vi "Value String to Details.vi"(9 "Datatype":T1, 10 "Default":variant, 11 "Value String":string) -> (2 "Identified?":bool, 3 "Value Variant":variant)   [LabVIEW 2016]
uses:
  data types/Datatype.ctl
  <userlib>/_OpenG.lib/lvdata/lvdata.llb/Type Descriptor Enumeration__ogtk.ctl
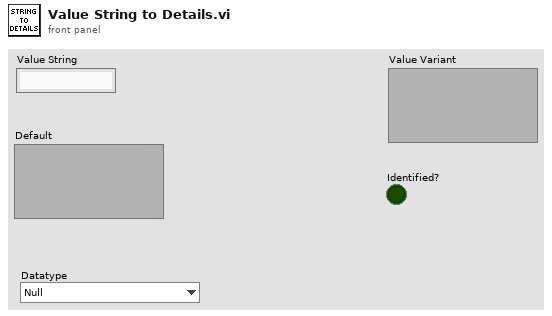
[diagram p1: front panel]
types:
  T1 = typedef "Datatype.ctl" = enum16{"Null", "Numeric", "String", "Bool", "Numeric 1D", "String 1D", "Bool 1D", "Numeric 2D", "String 2D", "Bool 2D", "Variant"}
  T2 = typedef "Type Descriptor Enumeration__ogtk.ctl" = enum8{"<Null>", "I8", "I16", "I32", "I64", "U8", "U16", "U32", "U64", "SGL", "DBL", "EXT", "CSG", "CDB", "CXT", "0x0F", "0x10", "0x11", "0x12", "0x13", "0x14", "Enum U8", "Enum U16", "Enum U32", "Enum U64", "SGL PQ", "DBL PQ", "EXT PQ", "CSG PQ", "CDB PQ", "CXT PQ", "0x1F", "0x20", "Boolean", "0x22", "0x23", "0x24", "0x25", "0x26", "0x27", "0x28", "0x29", "0x2A", "0x2B", "0x2C", "0x2D", "0x2E", "0x2F", "String", "0x31", "Path", "Pict", "0x34", "0x35", "0x36", "DAQ", "0x38", "0x39", "0x3A", "0x3B", "0x3C", "0x3D", "0x3E", "0x3F", "Array", "0x41", "0x42", "0x43", "0x44", "0x45", "0x46", "0x47", "0x48", "0x49", "0x4A", "0x4B", "0x4C", "0x4D", "0x4E", "0x4F", "Cluster", "0x51", "0x52", "Variant", "Waveform", "0x55", "0x56", "0x57", "0x58", "0x59", "0x5A", "0x5B", "0x5C", "0x5D", "0x5E", "0x5F", "0x60", "0x61", "0x62", "0x63", "0x64", "0x65", "0x66", "0x67", "0x68", "0x69", "0x6A", "0x6B", "0x6C", "0x6D", "0x6E", "0x6F", "Refnum"}
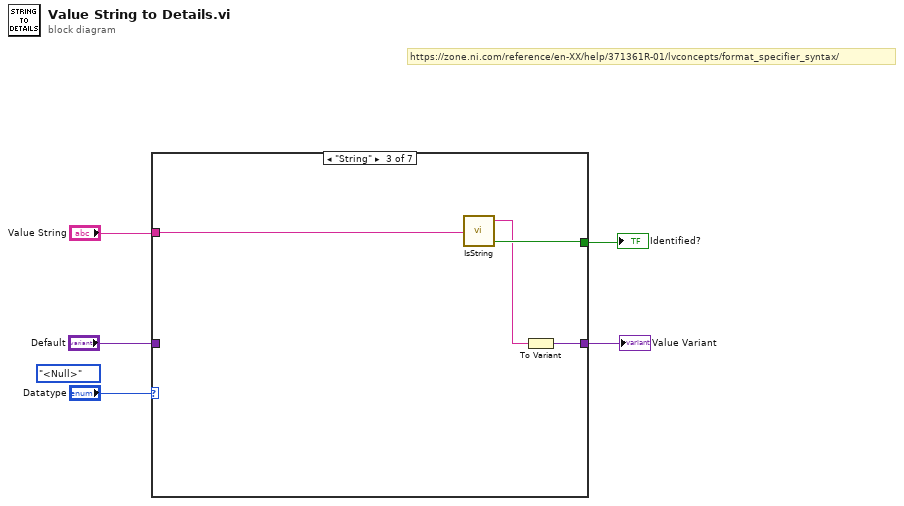
[diagram p0: block diagram]
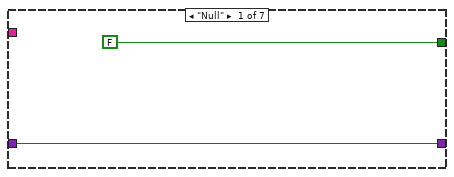
[diagram p2: hidden frame]
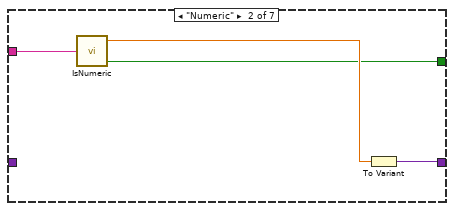
[diagram p3: hidden frame]
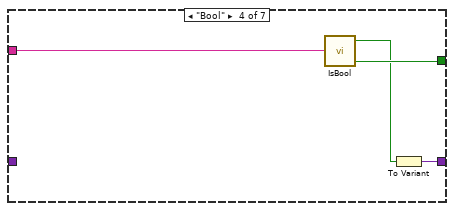
[diagram p4: hidden frame]
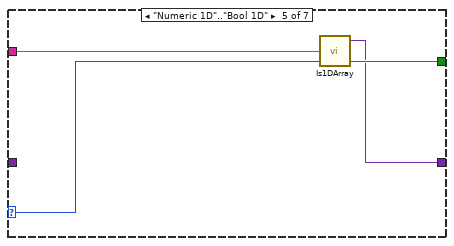
[diagram p5: hidden frame]
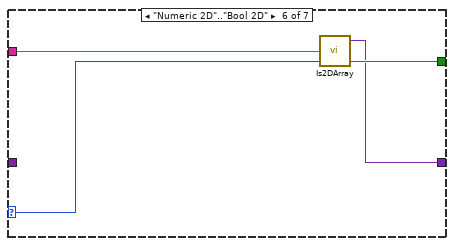
[diagram p6: hidden frame]
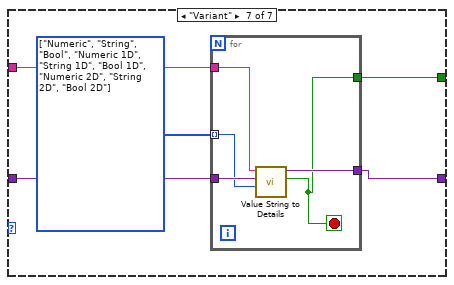
[diagram p7: hidden frame]
diagram:
  (unwired) Type_Descriptor_Enumeration__ogtk."<Null>" ("Type Descriptor Enumeration")
  # "https://zone.ni.com/reference/en-XX/help/371361R-01/lvconcepts/format_specifier_syntax/"
  n1 = case shown="\"String\"" "Datatype" {
    selector: "Datatype" -> [_ _ _ _ w21 w25 _]
    tunnel: "Value String" -> [_ w11 w15 w19 w23 w27 w32]
    tunnel: [w7 w8 w12 w17 w20 w24 w29] -> w3
    tunnel: "Default" -> [w7 _ _ _ _ _ w31]
    tunnel: [FALSE ("IsArray") w9 w14 w18 w22 w26 w28] -> w2
    frame "Null" {
    }
    frame "Numeric" {
      n2 = call "IsNumeric.vi"("Value String in"=w11) -> ("IsNumeric"=w9:bool, "Numeric Value"=w10:ext)  [unwired: 3 in]
      n3 = To Variant(anything=w10) -> (Variant=w8:variant)
    }
    frame "String" {
      n4 = call "IsString.vi"("Value String in"=w15) -> ("IsString"=w14:bool, "String Value"=w13:string)  [unwired: 3 in]
      n5 = To Variant(anything=w13) -> (Variant=w12:variant)
    }
    frame "Bool" {
      n6 = call "IsBool.vi"("Value String in"=w19) -> ("IsBool"=w18:bool, "Bool Value"=w16:bool)  [unwired: 3 in]
      n7 = To Variant(anything=w16) -> (Variant=w17:variant)
    }
    frame "Numeric 1D".."Bool 1D" {
      n8 = call "Is1DArray.vi"("Datatype"=w21, "Value String in"=w23) -> ("IsArray"=w22:bool, "Array Value"=w20:variant)  [unwired: 2 in]
    }
    frame "Numeric 2D".."Bool 2D" {
      n9 = call "Is2DArray.vi"("Datatype"=w25, "Value String in"=w27) -> ("IsArray"=w26:bool, "Array Value"=w24:variant)  [unwired: 2 in]
    }
    frame "Variant" {
      w30 = T1[] [enum."Numeric", enum."String", enum."Bool", enum."Numeric 1D", enum."String 1D", enum."Bool 1D", enum."Numeric 2D", enum."String 2D", enum."Bool 2D"] items=["Null", "Numeric", "String", "Bool", "Numeric 1D", "String 1D", "Bool 1D", "Numeric 2D", "String 2D", "Bool 2D", "Variant"]
      n10 = for {
        tunnel: w32 -> [w37]
        tunnel: w31 -> [w36]
        tunnel: [w35] -> w29
        tunnel: w30 -> [w34] mode=indexing
        tunnel: [w33] -> w28
        stop <- w33 stop-if-true
        n11 = call "Value String to Details.vi"("Datatype"=w34, "Default"=w36, "Value String"=w37) -> ("Identified?"=w33:bool, "Value Variant"=w35:variant)  [unwired: 7 in]
      }
    }
  }
  "Value Variant" <- w3
  "Identified?" <- w2
